vi "P4_p4 (1).vi"() -> ()   [LabVIEW 2024]
uses:
  <vilib>/Utility/file.llb/Write Delimited Spreadsheet (DBL).vi
panel:
  in  "Voltage Manual":dbl
  out "XY Graph":cluster{dbl[], dbl[]}(graph)
  out "RPM x 1000":dbl
  out "Waveform Chart":dynamicdata(graph)
  in  "Voltage":dbl(slide) scale=0.0..5.0
  out "Voltage Slide Level":dbl
  in  "stop":bool
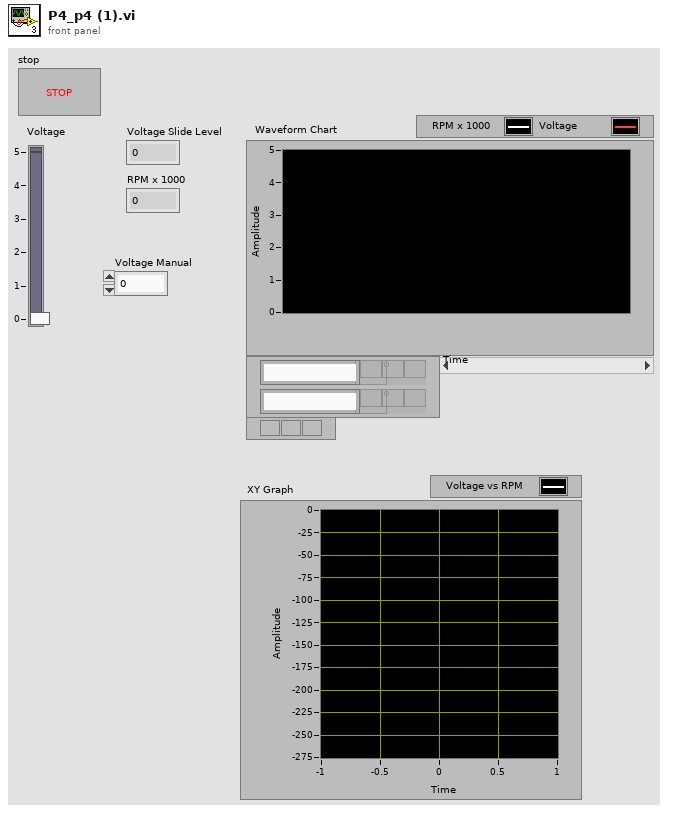
[diagram p1: front panel]
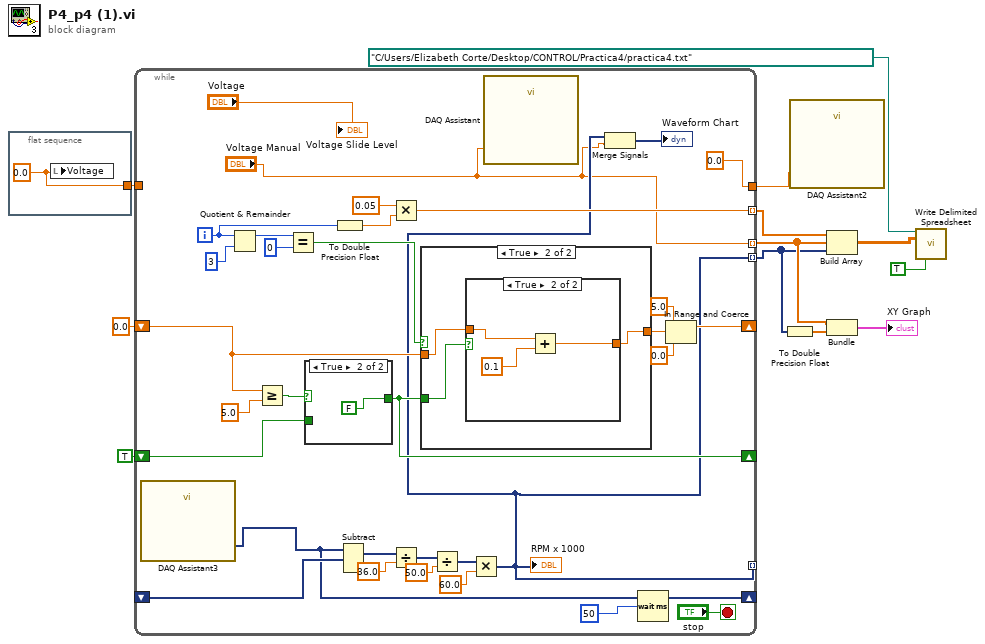
[diagram p0: block diagram]
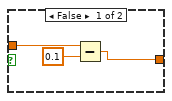
[diagram p3: hidden frame]
diagram:
  n1 = flat-sequence {
    tunnel: [w13] -> w12
    frame #0 {
      w13 = 0.0 ("Voltage")
      n2 = local write "Voltage"(w13) -> ()
    }
  }
  n3 = while {
    tunnel: w12 -> [_]
    shift-right: [w40] -> _
    shift-left: TRUE -> [w41]
    shift-right: [w18] -> _
    shift-left: 0.0 -> [w39]
    shift-right: [w14] -> _
    shift-left: _ -> [w27]
    tunnel: [w17] -> _ mode=indexing
    tunnel: [w20] -> w6 mode=indexing
    tunnel: ["Voltage Manual"] -> w5 mode=indexing
    tunnel: [w17] -> w2 mode=indexing
    tunnel: [0.0] -> w1
    i -> [w28]
    stop <- "stop" stop-if-true
    n4 = call "DAQ Assistant3"() -> ("data"=w14:dynamicdata)  [unwired: 16 in, 3 out]
    n5 = Quotient & Remainder(x=w28, y=3) -> (x-y*floor(x/y)=w37:i32)  [unwired: 1 out]
    n6 = Greater Or Equal?(x=w39, y=5.0) -> (x >= y?=w42:bool)
    n7 = Equal?(x=w37, y=0) -> (x = y?=w35:bool)
    n8 = case shown="True" w42 {
      tunnel: w41 -> [w56 _]
      tunnel: [w56 FALSE] -> w40
      frame False {
      }
      frame True {
      }
    }
    n9 = To Double Precision Float(number=w28) -> (double precision float=w29:dbl)
    n10 = Subtract(1:w27, 2:w14) -> (0:w26:dynamicdata)  [unwired: 1 in, 1 out]
    n11 = Multiply(x=0.05, y=w29) -> (x*y=w20:dbl)
    n12 = Divide(x=w26, y=36.0) -> (x/y=w24:dynamicdata)
    n13 = case shown="True" w35 {
      tunnel: w40 -> [_ w49]
      tunnel: w39 -> [w46 w48]
      tunnel: [w46 w47] -> w33
      frame False {
      }
      frame True {
        n14 = case shown="True" w49 {
          tunnel: w48 -> [w52 w55]
          tunnel: [w50 w53] -> w47
          frame False {
            n15 = Subtract(x=w52, y=0.1) -> (x-y=w50:dbl)
          }
          frame True {
            n16 = Add(x=w55, y=0.1) -> (x+y=w53:dbl)
          }
        }
      }
    }
    n17 = Divide(x=w24, y=50.0) -> (x/y=w22:dynamicdata)
    n18 = Multiply(x=w22, y=60.0) -> (x*y=w17:dynamicdata)
    "RPM x 1000" <- w17
    n19 = call "DAQ Assistant"("data"="Voltage Manual") -> ()  [unwired: 17 in, 2 out]
    n20 = Merge Signals(w17, "Voltage Manual") -> (→"Waveform Chart":dynamicdata)
    n21 = Wait (ms)(milliseconds to wait=u32 50) -> ()  [unwired: 1 out]
    n22 = In Range and Coerce(upper limit=5.0, x=w33, lower limit=0.0) -> (coerced(x)=w18:dbl)  [unwired: 1 out]
    "Voltage Slide Level" <- "Voltage"
  }
  n23 = To Double Precision Float(number=w2) -> (double precision float=w3:dbl[])
  n24 = call "DAQ Assistant2"("data"=w1) -> ()  [unwired: 17 in, 2 out]
  n25 = Build Array(w6, w5, w2) -> (w9:dbl[][])
  n26 = Bundle(w5, w3) -> (→"XY Graph":cluster{dbl[], dbl[]})  [unwired: 1 in]
  n27 = call-poly <vilib>:"Write Delimited Spreadsheet.vi"("file path (dialog if empty)"=path "C:/Users/Elizabeth Corte/Desktop/CONTROL/Practica4/practica4.txt", "2D data"=w9, "transpose? (no:F)"=TRUE) -> ()  [unwired: 11 in, 2 out]
